vi "WVDIAL_Main2.vi"() -> ()   [LabVIEW 2012]
uses:
  WVDIAL_GlobalVariables.vi
  TypeDefinitions.llb/TypeDef_LoopStagesMain.ctl
  TypeDefinitions.llb/TypeDef_ConfigureFIleTypes.ctl
  TypeDefinitions.llb/TypeDef_MainControlSystem.ctl
  TypeDefinitions.llb/TypeDef_ChildReporting.ctl
  <vilib>/Utility/miscctls.llb/LVRectTypeDef.ctl
  <vilib>/Utility/miscctls.llb/LVPointTypeDef.ctl
panel:
  out "FileUpdateTime":dbl
  out "WritePaths":path[](array[path])
  out "FileBaseNames":string[](array[string])
  out "DataBasePath":string="C:\\Users\\h2odial\\Desktop\\WVDCode\\WVD-MCSupdate\\WVDNewArchitectureUpdate\\WVD_Architecture_Update\\DataFolder"
  out "Children Responding":T2(array[cluster])
  out "QueueElement":string
  out "LoopCounter":i32
  out "Permission Level":T3(ring)
  in  "User Comment":bool
  in  "Update Permissions":bool
  in  "Global Abort":bool
  in  "Tab Control":T4(tab)
  in  "LaserLocking":bool
  in  "MCS":bool
  in  "Weather Station":bool
  in  "Template":bool
  in  "Operations":bool
  in  "Warmup":bool
  out "error IO":errorcluster
  out "SubPanelWidth":i32
  out "SubPanelHeight":i32
  out "What to Do":string
  in  "Software Testing":bool
  out "Pages":refnum<vi>[](array[refnum])
  out "SubPanelRefs":refnum<vi>[](array[refnum])
  # "Main Programs"
  # "Testing Programs"
  # "Individual Controls"
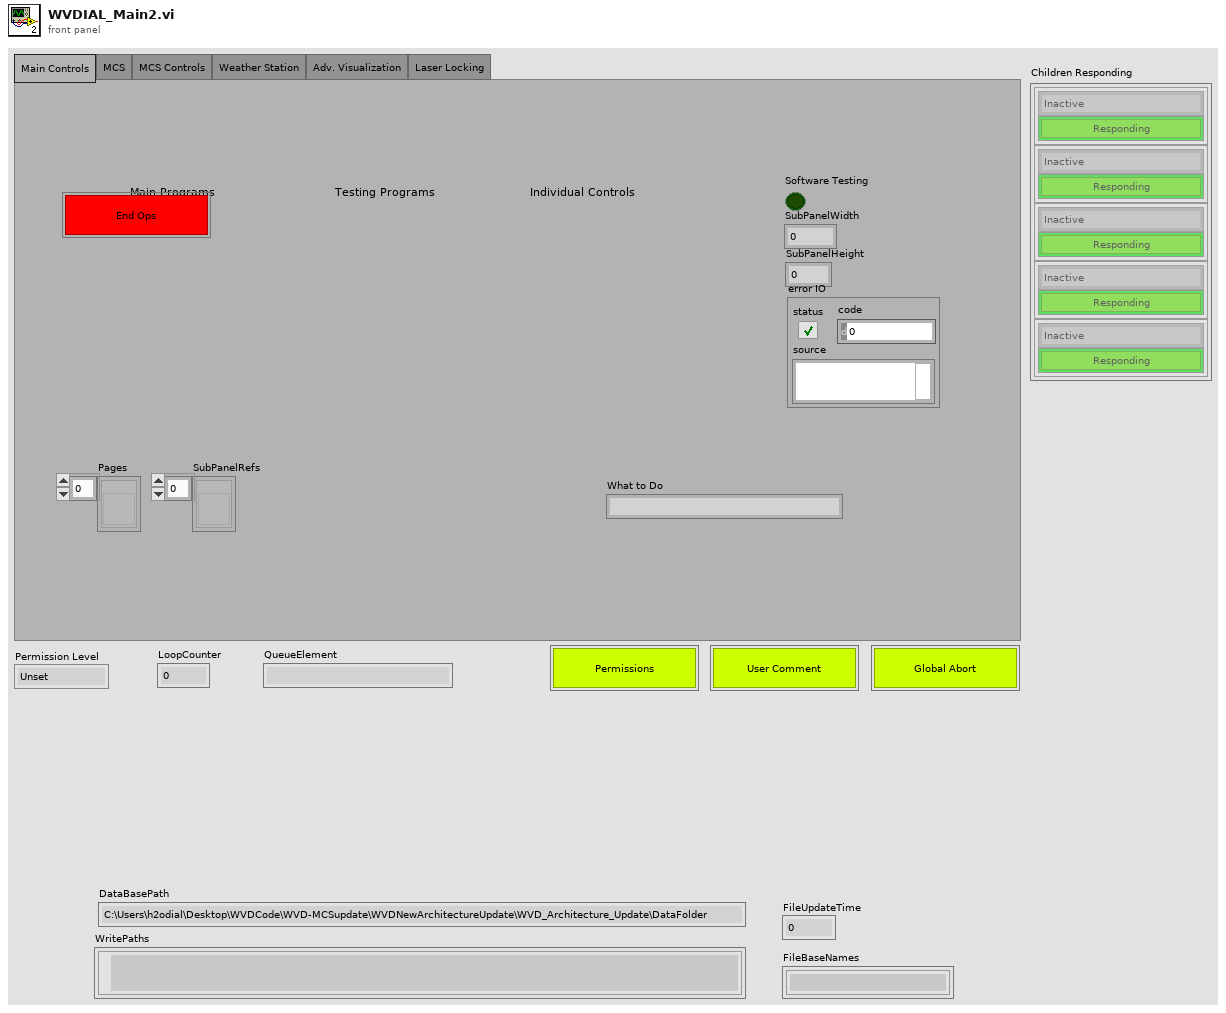
[diagram p1: front panel]
types:
  T1 = typedef "TypeDef_MainControlSystem.ctl" = enum16{"Inactive", "MCS", "MCSControls", "LaserControl", "LaserLocking", "WeatherStation", "DataDisplay", "Template", "WavelengthLocking"}
  T2 = cluster{"MainControlSystems":T1, "Responding":bool}[]
  T3 = enum16{"Unset", "Operator", "Administrator", "Full"}
  T4 = enum32{"Main Controls", "Inner Function 1", "Inner Function 2", "Inner Function 3", "Inner Function 4", "Inner Function 5", "Inner Function 6", "Inner Function 7", "Inner Function 8"}
  T5 = typedef "TypeDef_LoopStagesMain.ctl" = enum16{"Configure", "Initialize", "Idle", "ExitChildren", "Error Handler", "Exit"}
  T6 = typedef "LVPointTypeDef.ctl" = cluster{"Horizontal":i16, "Vertical":i16}
  T7 = typedef "LVRectTypeDef.ctl" = cluster{"Left":i16, "Top":i16, "Right":i16, "Bottom":i16}
  T8 = typedef "TypeDef_ConfigureFIleTypes.ctl" = enum16{"Main", "OpsMain", "OpsTemplate", "OpsWarmup", "OpsMCS", "OpsWeatherStation", "OpsWavlengthLocking", "ChildHousekeeping", "ChildLaserLocking", "ChildMCS", "ChildMCSControl", "ChildPowerSwitches", "ChildQuantumComposer", "ChildTemplate", "ChildUPS", "ChildWeatherStation", "ChildPlotting", "TestingSwitches", "TestingWavemeter"}
  T9 = typedef "TypeDef_ChildReporting.ctl" = cluster{"Child Command Stop":bool, "Child Responding":bool, "MainControlSystems":T1, "LastReportTime":dbl, "Child Exiting":bool}
  T10 = enum32{"Page Enabled", "Page Disabled", "Page Disabled & Grayed"}
  T11 = cluster{"MainControlSystems":T1, "Responding":bool}
  T12 = enum16{"Always On", "Always Off", "Off While Running"}
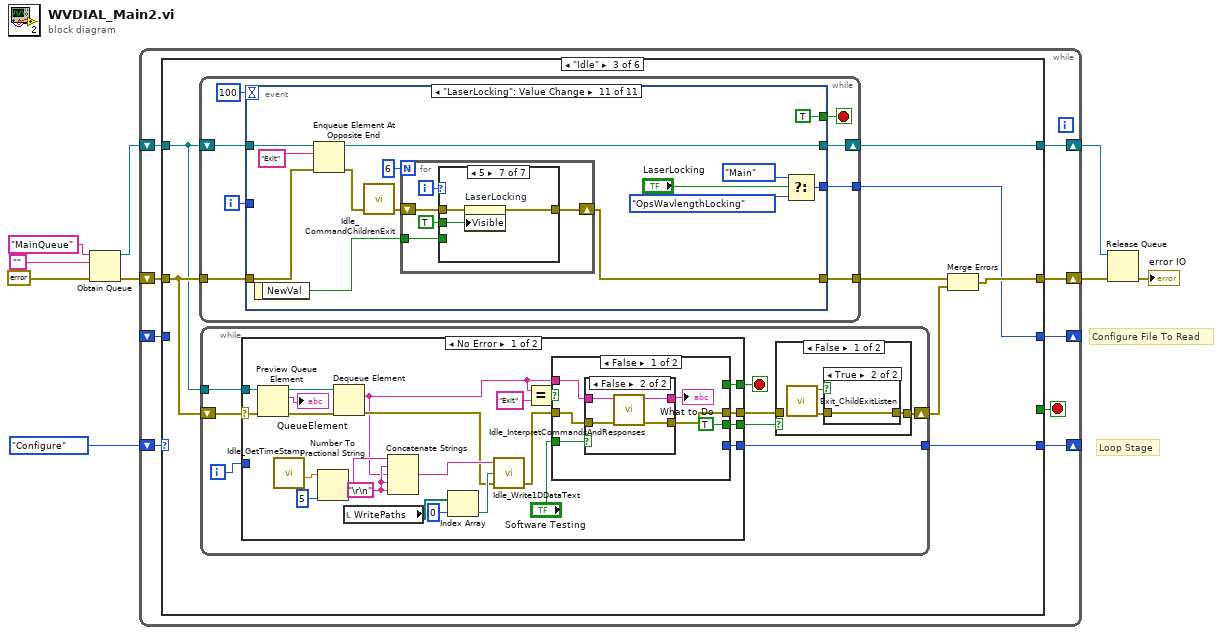
[diagram p0: block diagram]
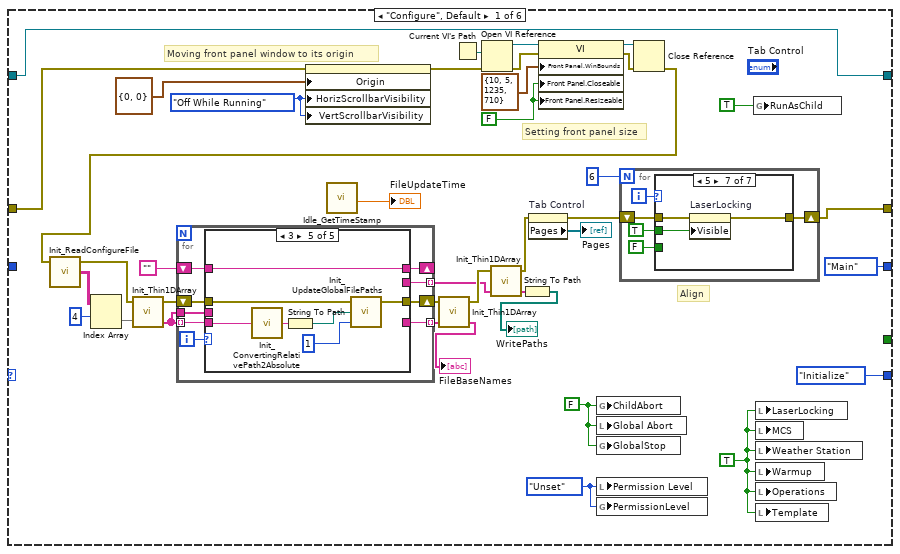
[diagram p2: hidden frame]
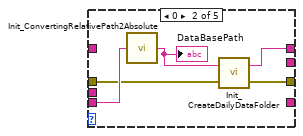
[diagram p4: hidden frame]
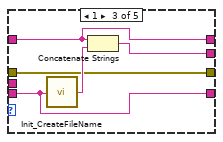
[diagram p5: hidden frame]
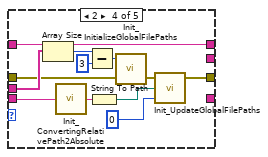
[diagram p6: hidden frame]
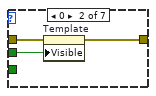
[diagram p8: hidden frame]
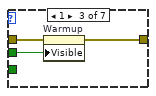
[diagram p9: hidden frame]
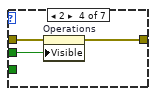
[diagram p10: hidden frame]
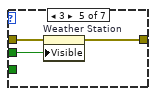
[diagram p11: hidden frame]
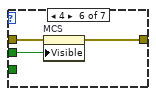
[diagram p12: hidden frame]
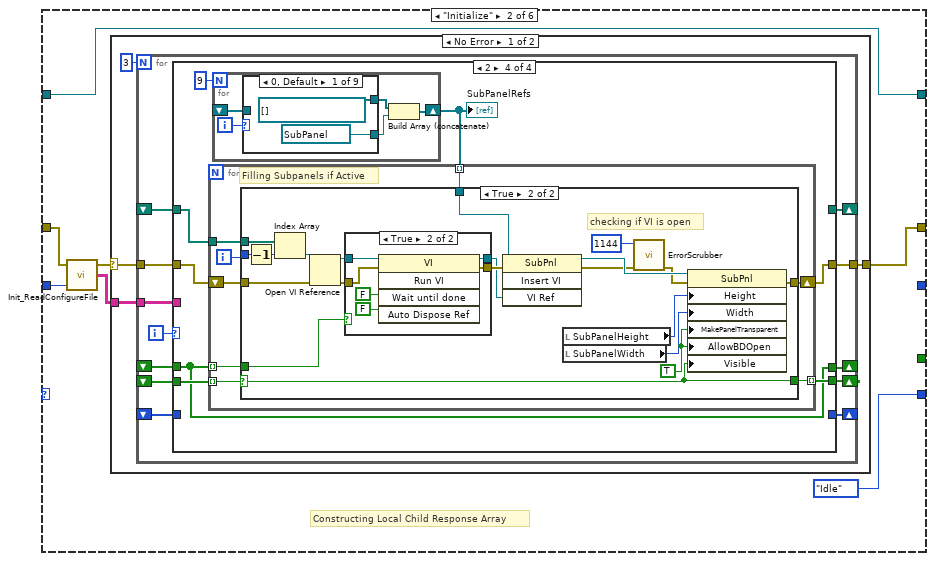
[diagram p13: hidden frame]
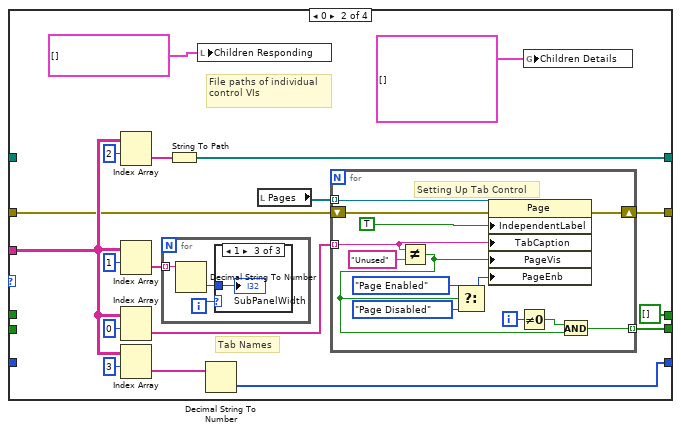
[diagram p15: hidden frame]
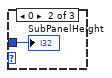
[diagram p17: hidden frame]
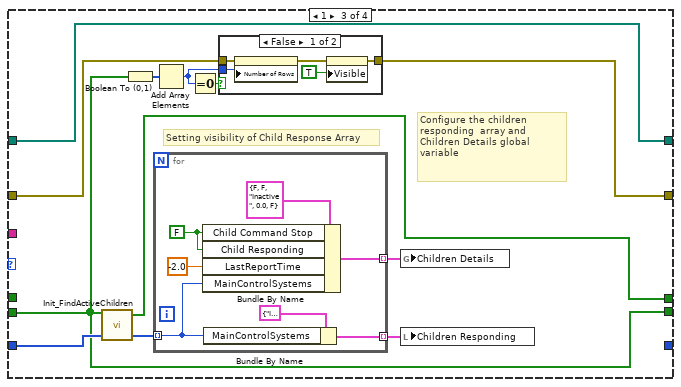
[diagram p18: hidden frame]
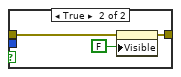
[diagram p19: hidden frame]
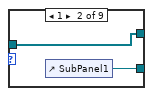
[diagram p20: hidden frame]
diagram:
  # "Configure File To Read"
  # "Loop Stage"
  n1 = Obtain Queue(name (unnamed)="MainQueue", element data type="", error in (no error)=errorcluster {"status"=FALSE, "code"=0, "source"=""}) -> (queue out=w3:refnum<queue>, error out=w4:errorcluster)  [unwired: 2 in, 1 out]
  n2 = while {
    shift-right: [w14] -> w7
    shift-left: w4 -> [w15]
    shift-right: [w13] -> w8
    shift-left: w3 -> [w12]
    shift-right: [w17] -> _
    shift-left: TypeDef_LoopStagesMain."Configure" ("Enum") -> [w18]
    shift-right: [w11] -> _
    shift-left: _ -> [w10]
    stop <- w16 stop-if-true
    n3 = case shown="\"Idle\"" w18 {
      tunnel: [TypeDef_LoopStagesMain."Initialize" ("Enum") TypeDef_LoopStagesMain."Idle" ("Enum") w288 TypeDef_LoopStagesMain."Initialize" ("Enum") TypeDef_LoopStagesMain."Idle" ("Enum") TypeDef_LoopStagesMain."Exit" ("Enum")] -> w17
      tunnel: [_ _ _ _ _ TRUE] -> w16
      tunnel: [w38 w127 w285 w646 w661 w667] -> w14
      tunnel: w15 -> [w40 w125 w289 w645 w661 w664]
      tunnel: [w41 w126 w290 w650 w659 w669] -> w13
      tunnel: w12 -> [w41 w126 w284 w650 w659 w669]
      tunnel: [TypeDef_ConfigureFIleTypes."Main" ("MainControlSystems") _ w283 w648 _ _] -> w11
      tunnel: w10 -> [_ w122 _ w648 _ _]
      frame "Configure", Default {
        w44 = T12."Off While Running" ("Vertical Scrollbar Visibility")
        w51 = FALSE
        w37 = TRUE ("Warmup")
        w52 = T3."Unset" ("Permission Level")
        w54 = FALSE ("Global Stop")
        # "Align"
        # "Setting front panel size"
        # "Moving front panel window to its origin"
        n4 = property on="Pane" class="Pane"(error in=w40, "Origin"=T6 {"Horizontal"=0, "Vertical"=0}, "HorizScrollbarVisibility"=w44, "VertScrollbarVisibility"=w44) -> (error out=w42:errorcluster)  [unwired: 1 in, 1 out]
        n5 = call "Idle_GetTimeStamp.vi"() -> ("Fractional Hours"=→"FileUpdateTime":dbl)  [unwired: 11 in]
        n6 = Current VI's Path() -> (path=w45:path)
        n7 = Open VI Reference(vi path=w45, error in (no error)=w42) -> (vi reference=w46:refnum<vi>, error out=w47:errorcluster)  [unwired: 4 in]
        n8 = property class="VI"(reference=w46, error in=w47, "Front Panel.WinBounds"=T7 {"Left"=10, "Top"=5, "Right"=1235, "Bottom"=710} ("Front Panel Window:Panel Bounds"), "Front Panel.Closeable"=w51, "Front Panel.Resizeable"=w51) -> (reference out=w48:refnum<vi>, error out=w49:errorcluster)
        n9 = global write "WVDIAL_GlobalVariables.vi" "ChildAbort"(w54) -> ()
        n10 = local write "Global Abort"(w54) -> ()
        n11 = global write "WVDIAL_GlobalVariables.vi" "GlobalStop"(w54) -> ()
        n12 = local write "Permission Level"(w52) -> ()
        n13 = global write "WVDIAL_GlobalVariables.vi" "PermissionLevel"(w52) -> ()
        n14 = Close Reference(reference=w48, error in (no error)=w49) -> (error out=w19:errorcluster)
        n15 = call "Init_ReadConfigureFile.vi"("error in"=w19) -> ("Parsed List"=w22:string[][], "error out"=w23:errorcluster)  [unwired: 2 in, 1 out]
        n16 = Index Array(array=w22, index (row)=4) -> (element=w26:string[])  [unwired: 1 in]
        n17 = call "Init_Thin1DArray.vi"("Padded Array"=w26, "ErrorIn"=w23) -> ("ThinnedArray"=w28:string[], "ErrorOut"=w27:errorcluster)  [unwired: 1 in, 1 out]
        n18 = for {
          shift-right: [w63] -> w30
          shift-left: w27 -> [w64]
          tunnel: w28 -> [w65] mode=indexing
          shift-right: [w62] -> _
          shift-left: "" -> [w61]
          tunnel: [w60] -> w31 mode=indexing
          tunnel: [w59] -> w34 mode=indexing
          tunnel: w28 -> [w58]
          i -> [w66]
          n19 = case shown="3" w66 {
            tunnel: w65 -> [_ w73 w75 w90 w97]
            tunnel: w64 -> [w67 w71 w77 w87 w95]
            tunnel: [w67 w70 w77 w86 w94] -> w63
            tunnel: [w68 w72 w76 w89 w96] -> w62
            tunnel: w61 -> [w68 _ w76 w89 w96]
            tunnel: [_ _ w75 _ _] -> w60
            tunnel: [_ _ w74 _ _] -> w59
            tunnel: w58 -> [_ _ _ w88 _]
            frame -1, Default {
            }
            frame 0 {
              n20 = call "Init_ConvertingRelativePath2Absolute.vi"("PathFromConfigureFileIn"=w73) -> ("PathOut"=w69:string)
              "DataBasePath" <- w69
              n21 = call "Init_CreateDailyDataFolder.vi"("ErrorIn"=w71, "PathIn"=w69) -> ("ErrorOut"=w70:errorcluster, "PathOut"=w72:string)
            }
            frame 1 {
              n22 = call "Init_CreateFileName.vi"("BaseFileName"=w75) -> ("FileName"=w78:string)
              n23 = Concatenate Strings(w76, w78) -> (w74:string)
            }
            frame 2 {
              n24 = Array Size(array=w88) -> (size(s)=w84:i32)
              n25 = call "Init_ConvertingRelativePath2Absolute.vi"("PathFromConfigureFileIn"=w90) -> ("PathOut"=w85:string)
              n26 = Subtract(x=w84, y=3) -> (x-y=w82:i32)
              n27 = String To Path(string=w85) -> (path=w81:path)
              n28 = call "Init_InitializeGlobalFilePaths.vi"("ErrorIn"=w87, "Entries"=w82) -> ("ErrorOut"=w80:errorcluster)  [unwired: 1 in]
              n29 = call "Init_UpdateGlobalFilePaths.vi"("PathIndex"=0, "NewPath"=w81, "ErrorIn"=w80) -> ("ErrorOut"=w86:errorcluster)  [unwired: 2 in]
            }
            frame 3 {
              n30 = call "Init_ConvertingRelativePath2Absolute.vi"("PathFromConfigureFileIn"=w97) -> ("PathOut"=w93:string)
              n31 = String To Path(string=w93) -> (path=w92:path)
              n32 = call "Init_UpdateGlobalFilePaths.vi"("PathIndex"=1, "NewPath"=w92, "ErrorIn"=w95) -> ("ErrorOut"=w94:errorcluster)  [unwired: 2 in]
            }
          }
        }
        n33 = call "Init_Thin1DArray.vi"("Padded Array"=w31, "ErrorIn"=w30) -> ("ThinnedArray"=→"FileBaseNames":string[], "ErrorOut"=w35:errorcluster)  [unwired: 1 in, 1 out]
        n34 = call "Init_Thin1DArray.vi"("Padded Array"=w34, "ErrorIn"=w35) -> ("ThinnedArray"=w32:string[], "ErrorOut"=w21:errorcluster)  [unwired: 1 in, 1 out]
        n35 = String To Path(string=w32) -> (path=→"WritePaths":path[])
        n36 = property on="Tab Control" class="TabCtl (strict)"(error in=w21) -> (error out=w39:errorcluster, "Pages"=→"Pages":refnum<vi>[])  [unwired: 1 in, 1 out]
        n37 = for {
          N: 6 -> [_]
          shift-right: [w100] -> w38
          shift-left: w39 -> [w101]
          i -> [w102]
          n38 = case shown="5" w102 {
            tunnel: w101 -> [w103 w106 w109 w112 w115 w117 w121]
            tunnel: [w103 w105 w108 w111 w114 w118 w120] -> w100
            tunnel: TRUE ("Visible") -> [_ w104 w107 w110 w113 w116 w119]
            tunnel: FALSE ("Visible") -> [_ _ _ _ _ _ _]
            frame -1, Default {
            }
            frame 0 {
              n39 = property on="Template" class="Bool (strict)"(error in=w106, "Visible"=w104) -> (error out=w105:errorcluster)  [unwired: 1 in, 1 out]
            }
            frame 1 {
              n40 = property on="Warmup" class="Bool (strict)"(error in=w109, "Visible"=w107) -> (error out=w108:errorcluster)  [unwired: 1 in, 1 out]
            }
            frame 2 {
              n41 = property on="Operations" class="Bool (strict)"(error in=w112, "Visible"=w110) -> (error out=w111:errorcluster)  [unwired: 1 in, 1 out]
            }
            frame 3 {
              n42 = property on="Weather Station" class="Bool (strict)"(error in=w115, "Visible"=w113) -> (error out=w114:errorcluster)  [unwired: 1 in, 1 out]
            }
            frame 4 {
              n43 = property on="MCS" class="Bool (strict)"(error in=w117, "Visible"=w116) -> (error out=w118:errorcluster)  [unwired: 1 in, 1 out]
            }
            frame 5 {
              n44 = property on="LaserLocking" class="Bool (strict)"(error in=w121, "Visible"=w119) -> (error out=w120:errorcluster)  [unwired: 1 in, 1 out]
            }
          }
        }
        n45 = global write "WVDIAL_GlobalVariables.vi" "RunAsChild"(TRUE ("RunAsChild")) -> ()
        n46 = local write "LaserLocking"(w37) -> ()
        n47 = local write "MCS"(w37) -> ()
        n48 = local write "Weather Station"(w37) -> ()
        n49 = local write "Warmup"(w37) -> ()
        n50 = local write "Operations"(w37) -> ()
        n51 = local write "Template"(w37) -> ()
      }
      frame "Initialize" {
        # "Constructing Local Child Response Array"
        n52 = call "Init_ReadConfigureFile.vi"("ConfigureFileType"=w122, "error in"=w125) -> ("Parsed List"=w123:string[][], "error out"=w124:errorcluster)  [unwired: 1 in, 1 out]
        n53 = case shown="No Error" w124 {
          selector: w124 -> [w131 w282]
          tunnel: [w132 w282] -> w127
          tunnel: w123 -> [w130 _]
          frame No Error {
            n54 = for {
              N: 3 -> [_]
              tunnel: [w144] -> w132
              tunnel: w131 -> [w137]
              tunnel: w130 -> [w142]
              shift-right: [w141] -> _
              shift-left: _ -> [w140]
              shift-right: [w139] -> _
              shift-left: _ -> [w138]
              shift-right: [w136] -> _
              shift-left: _ -> [w135]
              shift-right: [w134] -> _
              shift-left: _ -> [w133]
              i -> [w143]
              n55 = case shown="2" w143 {
                tunnel: [w148 w159 w194 w220] -> w144
                tunnel: w137 -> [w148 w151 w195 w217]
                tunnel: w142 -> [_ w157 _ _]
                tunnel: [w149 w163 w188 _] -> w141
                tunnel: w140 -> [w149 _ w188 w219]
                tunnel: [w147 w160 w190 w216] -> w139
                tunnel: w138 -> [w147 _ w190 w218]
                tunnel: [w146 w155 _ _] -> w136
                tunnel: w135 -> [w146 _ w191 _]
                tunnel: [w145 bool[] [] ("StartSubVI") w186 w213] -> w134
                tunnel: w133 -> [w145 _ _ w213]
                frame -1, Default {
                }
                frame 0 {
                  # "File paths of individual control VIs"
                  # "Tab Names"
                  n56 = Index Array(array=w157, index (row)=2) -> (element=w164:string[])  [unwired: 1 in]
                  n57 = Index Array(array=w157, index (row)=1) -> (element=w162:string[])  [unwired: 1 in]
                  n58 = Index Array(array=w157, index (row)=0) -> (element=w161:string[])  [unwired: 1 in]
                  n59 = Index Array(array=w157, index (row)=3) -> (element=w156:string[])  [unwired: 1 in]
                  n60 = for {
                    tunnel: w162 -> [w182] mode=indexing
                    i -> [w183]
                    n61 = Decimal String To Number(string=w182) -> (number=w181:i32)  [unwired: 2 in, 1 out]
                    n62 = case shown="1" w183 {
                      tunnel: w181 -> [_ w184 w185]
                      frame -1, Default {
                      }
                      frame 0 {
                        "SubPanelHeight" <- w184
                      }
                      frame 1 {
                        "SubPanelWidth" <- w185
                      }
                    }
                  }
                  n63 = String To Path(string=w164) -> (path=w163:path[])
                  n64 = local write "Children Responding"(T2 [] ("Children Responding")) -> ()
                  n65 = Decimal String To Number(string=w156) -> (number=w155:i32[])  [unwired: 2 in, 1 out]
                  n66 = local read "Pages"() -> (w152:refnum<vi>[])
                  n67 = for {
                    tunnel: w161 -> [w174] mode=indexing
                    tunnel: w152 -> [w177] mode=indexing
                    shift-right: [w175] -> w159
                    shift-left: w151 -> [w176]
                    tunnel: [w171] -> w160 mode=indexing
                    i -> [w172]
                    # "Setting Up Tab Control"
                    n68 = Not Equal?(x=w174, y="Unused") -> (x != y?=w169:bool)
                    n69 = Select(t=T10."Page Enabled" ("Page Enabled State"), s=w169, f=T10."Page Disabled" ("Page Enabled State")) -> (s? t:f=w168:T10)
                    n70 = property class="Page"(reference=w177, error in=w176, "IndependentLabel"=TRUE ("Independent Label"), "TabCaption"=w174, "PageVis"=w169, "PageEnb"=w168) -> (error out=w175:errorcluster)  [unwired: 1 out]
                    n71 = Not Equal To 0?(x=w172) -> (x != 0?=w173:bool)
                    n72 = And(x=w173, y=w169) -> (x .and. y?=w171:bool)
                  }
                  n73 = global write "WVDIAL_GlobalVariables.vi" "Children Details"(T9[] []) -> ()
                }
                frame 1 {
                  # "Setting visibility of Child Response Array"
                  # "Configure the children responding  array and Children Details global variable"
                  n74 = call "Init_FindActiveChildren.vi"("ChannelType"=w191, "ChannelOn"=w190) -> ("ActiveTypes"=w189:i32[], "StartSubVI"=w186:bool[])  [unwired: 1 in, 1 out]
                  n75 = Boolean To (0,1)(Boolean=w190) -> (0, 1=w197:i16[])
                  n76 = for {
                    tunnel: [w211] -> w196 mode=indexing
                    tunnel: w189 -> [w206] mode=indexing
                    tunnel: [w209] -> w187 mode=indexing
                    w208 = FALSE
                    n77 = Bundle By Name(cluster=T9 {"Child Command Stop"=FALSE, "Child Responding"=FALSE, "MainControlSystems"=enum."Inactive", "LastReportTime"=0.0, "Child Exiting"=FALSE} ("Child Details"), "Child Command Stop"=w208, "Child Responding"=w208, "LastReportTime"=-2.0, "MainControlSystems"=w206) -> (w209:T9)
                    n78 = Bundle By Name(cluster=T11 {"MainControlSystems"=enum."Inactive", "Responding"=TRUE} ("ChildResponse"), "MainControlSystems"=w206) -> (w211:T11)
                  }
                  n79 = Add Array Elements(numeric array=w197) -> (sum=w193:i16)
                  n80 = Equal To 0?(x=w193) -> (x = 0?=w192:bool)
                  n81 = case shown="False" w192 {
                    tunnel: w195 -> [w202 w205]
                    tunnel: [w199 w204] -> w194
                    tunnel: w193 -> [w201 _]
                    frame False {
                      n82 = property on="Children Responding" class="Arr (strict)"(error in=w202, "Number of Rows"=w201) -> (error out=w200:errorcluster)  [unwired: 1 in, 1 out]
                      n83 = property on="Children Responding" class="Arr (strict)"(error in=w200, "Visible"=TRUE) -> (error out=w199:errorcluster)  [unwired: 1 in, 1 out]
                    }
                    frame True {
                      n84 = property on="Children Responding" class="Arr (strict)"(error in=w205, "Visible"=FALSE) -> (error out=w204:errorcluster)  [unwired: 1 in, 1 out]
                    }
                  }
                  n85 = global write "WVDIAL_GlobalVariables.vi" "Children Details"(w187) -> ()
                  n86 = local write "Children Responding"(w196) -> ()
                }
                frame 2 {
                  n87 = for {
                    N: 9 -> [_]
                    shift-right: [w225] -> w214
                    shift-left: _ -> [w221]
                    i -> [w224]
                    n88 = case shown="0, Default" w224 {
                      tunnel: [refnum<vi> refnum ("SubPanel8") w229 w231 w233 w235 w237 w239 w241 w243] -> w223
                      tunnel: [refnum<vi>[] [] w228 w230 w232 w234 w236 w238 w240 w242] -> w222
                      tunnel: w221 -> [_ w228 w230 w232 w234 w236 w238 w240 w242]
                      frame 0, Default {
                      }
                      frame 1 {
                        n89 = control-ref of="SubPanel1"() -> (w229:refnum<vi>)
                      }
                      frame 2 {
                        n90 = control-ref of="SubPanel2"() -> (w231:refnum<vi>)
                      }
                      frame 3 {
                        n91 = control-ref of="SubPanel3"() -> (w233:refnum<vi>)
                      }
                      frame 4 {
                        n92 = control-ref of="SubPanel4"() -> (w235:refnum<vi>)
                      }
                      frame 5 {
                        n93 = control-ref of="SubPanel5"() -> (w237:refnum<vi>)
                      }
                      frame 6 {
                        n94 = control-ref of="SubPanel6"() -> (w239:refnum<vi>)
                      }
                      frame 7 {
                        n95 = control-ref of="SubPanel7"() -> (w241:refnum<vi>)
                      }
                      frame 8 {
                        n96 = control-ref of="SubPanel8"() -> (w243:refnum<vi>)
                      }
                    }
                    n97 = Build Array (concatenate)(w222, w223) -> (w225:refnum<vi>[])
                  }
                  "SubPanelRefs" <- w214
                  n98 = for {
                    shift-right: [w250] -> w220
                    shift-left: w217 -> [w251]
                    tunnel: w219 -> [w249]
                    tunnel: w218 -> [w246] mode=indexing
                    tunnel: [w248] -> w216 mode=indexing
                    tunnel: w214 -> [w245] mode=indexing
                    tunnel: w213 -> [w244] mode=indexing
                    i -> [w247]
                    # "Filling Subpanels if Active"
                    n99 = case shown="True" w246 {
                      selector: w246 -> [w252 w258]
                      tunnel: w251 -> [w253 w273]
                      tunnel: [w253 w260] -> w250
                      tunnel: w249 -> [_ w272]
                      tunnel: w247 -> [_ w264]
                      tunnel: [w252 w258] -> w248
                      tunnel: w245 -> [_ w261]
                      tunnel: w244 -> [_ w257]
                      frame False {
                      }
                      frame True {
                        w265 = TRUE ("Allow User to Open Diagram")
                        # "checking if VI is open"
                        n100 = Decrement(x=w264) -> (x-1=w263:i32)
                        n101 = Index Array(array=w272, index=w263) -> (element=w271:path)
                        n102 = Open VI Reference(vi path=w271, error in (no error)=w273) -> (vi reference=w270:refnum<vi>, error out=w269:errorcluster)  [unwired: 4 in]
                        n103 = case shown="True" w257 {
                          tunnel: w270 -> [w275 w281]
                          tunnel: w269 -> [w274 w280]
                          tunnel: [w274 w278] -> w268
                          tunnel: [w275 w276] -> w259
                          frame False {
                          }
                          frame True {
                            n104 = invoke class="VI" method="Run VI"(reference=w281, error in=w280, "Wait until done"=FALSE ("Wait Until Done"), "Auto Dispose Ref"=FALSE ("Auto Dispose Reference")) -> (reference out=w276:refnum<vi>, error out=w278:errorcluster)  [unwired: 1 in, 3 out]
                          }
                        }
                        n105 = invoke on="Invoke Node" class="SubPnl" method="Insert VI"(reference=w261, error in=w268, "VI Ref"=w259) -> (reference out=w262:refnum<vi>, error out=w255:errorcluster)  [unwired: 1 in, 2 out]
                        n106 = local read "SubPanelHeight"() -> (w267:i32)
                        n107 = local read "SubPanelWidth"() -> (w266:i32)
                        n108 = call "ErrorScrubber.vi"("error in (no error)"=w255, "y"=1144) -> ("error out"=w256:errorcluster)  [unwired: 9 in]
                        n109 = property on="Property Node" class="SubPnl"(reference=w262, error in=w256, "Height"=w267, "Width"=w266, "MakePanelTransparent"=w265, "AllowBDOpen"=w265, "Visible"=w258) -> (error out=w260:errorcluster)  [unwired: 1 out]
                      }
                    }
                  }
                }
              }
            }
          }
          frame Error {
          }
        }
      }
      frame "Idle" {
        n110 = while {
          tunnel: w289 -> [w355]
          shift-right: [w350] -> w290
          shift-left: w284 -> [w351]
          tunnel: [w349] -> w286
          tunnel: [w348] -> w283
          i -> [w352]
          stop <- w353 stop-if-true
          n111 = event shown="[10] \"LaserLocking\": Value Change" {
            selector: _ -> [_ _ _ _ _ _ _ _ _ _ _]
            dyn-events: _ -> [_ _ _ _ _ _ _ _ _ _ _]
            timeout: 100 -> [_ _ _ _ _ _ _ _ _ _ _]
            tunnel: w355 -> [w362 w364 w370 w374 w389 w427 w466 w504 w542 w580 w618]
            tunnel: [_ "Global Abort" _ _ TRUE ("Global Abort") TRUE ("Global Abort") TRUE ("Global Abort") TRUE ("Global Abort") TRUE ("Global Abort") TRUE ("Global Abort") TRUE ("Global Abort")] -> w353
            tunnel: w352 -> [w361 _ _ _ _ _ _ _ _ _ _]
            tunnel: w351 -> [w360 w367 w373 w377 w391 w429 w468 w506 w544 w582 w620]
            tunnel: [w360 w366 w372 w376 w390 w428 w467 w505 w543 w581 w619] -> w350
            tunnel: [w362 w363 w369 w375 w380 w419 w460 w498 w536 w574 w612] -> w349
            tunnel: [_ _ _ _ w392 w430 w458 w496 w534 w572 w610] -> w348
            event Timeout {
              n112 = event-data() -> ()  [unwired: 1 in, 1 out]
              n113 = global read "WVDIAL_GlobalVariables.vi" "PermissionLevel"() -> (→"Permission Level":i32)
              n114 = local read "Children Responding"() -> (w357:T2)
              n115 = call "Idle_MainIdleProcess.vi"("ChildrenResponding"=w357) -> ("ChildrenDetailsUpdated"=w359:T9[], "ChildrenResponding"=→"Children Responding":T2)  [unwired: 1 in]
              n116 = global write "WVDIAL_GlobalVariables.vi" "Children Details"(w359) -> ()
              "LoopCounter" <- w361
            }
            event "Global Abort": Value Change {
              n117 = event-data() -> ()  [unwired: 1 in, 1 out]
              n118 = Enqueue Element At Opposite End(queue=w367, element="Exit", error in (no error)=w364) -> (queue out=w366:refnum<queue>, error out=w363:errorcluster)  [unwired: 1 in, 1 out]
              n119 = global write "WVDIAL_GlobalVariables.vi" "GlobalStop"("Global Abort") -> ()
            }
            event "Update Permissions": Value Change {
              n120 = event-data() -> ()  [unwired: 1 in, 1 out]
              n121 = Enqueue Element(queue=w373, element="System_OpenPermissionsVI", error in (no error)=w370) -> (queue out=w372:refnum<queue>, error out=w369:errorcluster)  [unwired: 1 in, 1 out]
            }
            event "User Comment": Value Change {
              n122 = event-data() -> ()  [unwired: 1 in, 1 out]
              n123 = Enqueue Element(queue=w377, element="System_OpenUserCommentVI", error in (no error)=w374) -> (queue out=w376:refnum<queue>, error out=w375:errorcluster)  [unwired: 1 in, 1 out]
            }
            event "Template": Value Change {
              n124 = event-data() -> ("NewVal"=w379:bool)  [unwired: 1 in]
              n125 = Enqueue Element At Opposite End(queue=w391, element="Exit", error in (no error)=w389) -> (queue out=w390:refnum<queue>, error out=w384:errorcluster)  [unwired: 1 in, 1 out]
              n126 = call "Idle_CommandChildrenExit.vi"("ErrorIn"=w384) -> ("ErrorOut"=w381:errorcluster)  [unwired: 4 in]
              n127 = for {
                N: 6 -> [_]
                shift-right: [w395] -> w380
                shift-left: w381 -> [w396]
                tunnel: w379 -> [w393]
                i -> [w397]
                n128 = case shown="0" w397 {
                  tunnel: w396 -> [w398 w401 w404 w407 w410 w412 w416]
                  tunnel: [w398 w400 w403 w406 w409 w413 w415] -> w395
                  tunnel: TRUE ("Visible") -> [_ w399 _ _ _ _ _]
                  tunnel: w393 -> [_ _ w402 w405 w408 w411 w414]
                  frame -1, Default {
                  }
                  frame 0 {
                    n129 = property on="Template" class="Bool (strict)"(error in=w401, "Visible"=w399) -> (error out=w400:errorcluster)  [unwired: 1 in, 1 out]
                  }
                  frame 1 {
                    n130 = property on="Warmup" class="Bool (strict)"(error in=w404, "Visible"=w402) -> (error out=w403:errorcluster)  [unwired: 1 in, 1 out]
                  }
                  frame 2 {
                    n131 = property on="Operations" class="Bool (strict)"(error in=w407, "Visible"=w405) -> (error out=w406:errorcluster)  [unwired: 1 in, 1 out]
                  }
                  frame 3 {
                    n132 = property on="Weather Station" class="Bool (strict)"(error in=w410, "Visible"=w408) -> (error out=w409:errorcluster)  [unwired: 1 in, 1 out]
                  }
                  frame 4 {
                    n133 = property on="MCS" class="Bool (strict)"(error in=w412, "Visible"=w411) -> (error out=w413:errorcluster)  [unwired: 1 in, 1 out]
                  }
                  frame 5 {
                    n134 = property on="LaserLocking" class="Bool (strict)"(error in=w416, "Visible"=w414) -> (error out=w415:errorcluster)  [unwired: 1 in, 1 out]
                  }
                }
              }
              n135 = Select(t=TypeDef_ConfigureFIleTypes."Main" ("MainControlSystems"), s="Template", f=TypeDef_ConfigureFIleTypes."OpsTemplate" ("MainControlSystems")) -> (s? t:f=w392:T8)
            }
            event "Warmup": Value Change {
              n136 = event-data() -> ("NewVal"=w418:bool)  [unwired: 1 in]
              n137 = Enqueue Element At Opposite End(queue=w429, element="Exit", error in (no error)=w427) -> (queue out=w428:refnum<queue>, error out=w423:errorcluster)  [unwired: 1 in, 1 out]
              n138 = call "Idle_CommandChildrenExit.vi"("ErrorIn"=w423) -> ("ErrorOut"=w420:errorcluster)  [unwired: 4 in]
              n139 = for {
                N: 6 -> [_]
                shift-right: [w433] -> w419
                shift-left: w420 -> [w434]
                tunnel: w418 -> [w431]
                i -> [w435]
                n140 = case shown="5" w435 {
                  tunnel: w434 -> [w436 w439 w442 w445 w448 w450 w454]
                  tunnel: [w436 w438 w441 w444 w447 w451 w453] -> w433
                  tunnel: TRUE ("Visible") -> [_ _ w440 _ _ _ _]
                  tunnel: w431 -> [_ w437 _ w443 w446 w449 w452]
                  frame -1, Default {
                  }
                  frame 0 {
                    n141 = property on="Template" class="Bool (strict)"(error in=w439, "Visible"=w437) -> (error out=w438:errorcluster)  [unwired: 1 in, 1 out]
                  }
                  frame 1 {
                    n142 = property on="Warmup" class="Bool (strict)"(error in=w442, "Visible"=w440) -> (error out=w441:errorcluster)  [unwired: 1 in, 1 out]
                  }
                  frame 2 {
                    n143 = property on="Operations" class="Bool (strict)"(error in=w445, "Visible"=w443) -> (error out=w444:errorcluster)  [unwired: 1 in, 1 out]
                  }
                  frame 3 {
                    n144 = property on="Weather Station" class="Bool (strict)"(error in=w448, "Visible"=w446) -> (error out=w447:errorcluster)  [unwired: 1 in, 1 out]
                  }
                  frame 4 {
                    n145 = property on="MCS" class="Bool (strict)"(error in=w450, "Visible"=w449) -> (error out=w451:errorcluster)  [unwired: 1 in, 1 out]
                  }
                  frame 5 {
                    n146 = property on="LaserLocking" class="Bool (strict)"(error in=w454, "Visible"=w452) -> (error out=w453:errorcluster)  [unwired: 1 in, 1 out]
                  }
                }
              }
              n147 = Select(t=TypeDef_ConfigureFIleTypes."Main" ("MainControlSystems"), s="Warmup", f=TypeDef_ConfigureFIleTypes."OpsWarmup" ("MainControlSystems")) -> (s? t:f=w430:T8)
            }
            event "Operations": Value Change {
              n148 = event-data() -> ("NewVal"=w459:bool)  [unwired: 1 in]
              n149 = Enqueue Element At Opposite End(queue=w468, element="Exit", error in (no error)=w466) -> (queue out=w467:refnum<queue>, error out=w464:errorcluster)  [unwired: 1 in, 1 out]
              n150 = call "Idle_CommandChildrenExit.vi"("ErrorIn"=w464) -> ("ErrorOut"=w461:errorcluster)  [unwired: 4 in]
              n151 = for {
                N: 6 -> [_]
                shift-right: [w471] -> w460
                shift-left: w461 -> [w472]
                tunnel: w459 -> [w469]
                i -> [w473]
                n152 = case shown="5" w473 {
                  tunnel: w472 -> [w474 w477 w480 w483 w486 w488 w492]
                  tunnel: [w474 w476 w479 w482 w485 w489 w491] -> w471
                  tunnel: TRUE ("Visible") -> [_ _ _ w481 _ _ _]
                  tunnel: w469 -> [_ w475 w478 _ w484 w487 w490]
                  frame -1, Default {
                  }
                  frame 0 {
                    n153 = property on="Template" class="Bool (strict)"(error in=w477, "Visible"=w475) -> (error out=w476:errorcluster)  [unwired: 1 in, 1 out]
                  }
                  frame 1 {
                    n154 = property on="Warmup" class="Bool (strict)"(error in=w480, "Visible"=w478) -> (error out=w479:errorcluster)  [unwired: 1 in, 1 out]
                  }
                  frame 2 {
                    n155 = property on="Operations" class="Bool (strict)"(error in=w483, "Visible"=w481) -> (error out=w482:errorcluster)  [unwired: 1 in, 1 out]
                  }
                  frame 3 {
                    n156 = property on="Weather Station" class="Bool (strict)"(error in=w486, "Visible"=w484) -> (error out=w485:errorcluster)  [unwired: 1 in, 1 out]
                  }
                  frame 4 {
                    n157 = property on="MCS" class="Bool (strict)"(error in=w488, "Visible"=w487) -> (error out=w489:errorcluster)  [unwired: 1 in, 1 out]
                  }
                  frame 5 {
                    n158 = property on="LaserLocking" class="Bool (strict)"(error in=w492, "Visible"=w490) -> (error out=w491:errorcluster)  [unwired: 1 in, 1 out]
                  }
                }
              }
              n159 = Select(t=TypeDef_ConfigureFIleTypes."Main" ("MainControlSystems"), s="Operations", f=TypeDef_ConfigureFIleTypes."OpsMain" ("MainControlSystems")) -> (s? t:f=w458:T8)
            }
            event "Weather Station": Value Change {
              n160 = event-data() -> ("NewVal"=w497:bool)  [unwired: 1 in]
              n161 = Enqueue Element At Opposite End(queue=w506, element="Exit", error in (no error)=w504) -> (queue out=w505:refnum<queue>, error out=w502:errorcluster)  [unwired: 1 in, 1 out]
              n162 = call "Idle_CommandChildrenExit.vi"("ErrorIn"=w502) -> ("ErrorOut"=w499:errorcluster)  [unwired: 4 in]
              n163 = for {
                N: 6 -> [_]
                shift-right: [w509] -> w498
                shift-left: w499 -> [w510]
                tunnel: w497 -> [w507]
                i -> [w511]
                n164 = case shown="5" w511 {
                  tunnel: w510 -> [w512 w515 w518 w521 w524 w526 w530]
                  tunnel: [w512 w514 w517 w520 w523 w527 w529] -> w509
                  tunnel: TRUE ("Visible") -> [_ _ _ _ w522 _ _]
                  tunnel: w507 -> [_ w513 w516 w519 _ w525 w528]
                  frame -1, Default {
                  }
                  frame 0 {
                    n165 = property on="Template" class="Bool (strict)"(error in=w515, "Visible"=w513) -> (error out=w514:errorcluster)  [unwired: 1 in, 1 out]
                  }
                  frame 1 {
                    n166 = property on="Warmup" class="Bool (strict)"(error in=w518, "Visible"=w516) -> (error out=w517:errorcluster)  [unwired: 1 in, 1 out]
                  }
                  frame 2 {
                    n167 = property on="Operations" class="Bool (strict)"(error in=w521, "Visible"=w519) -> (error out=w520:errorcluster)  [unwired: 1 in, 1 out]
                  }
                  frame 3 {
                    n168 = property on="Weather Station" class="Bool (strict)"(error in=w524, "Visible"=w522) -> (error out=w523:errorcluster)  [unwired: 1 in, 1 out]
                  }
                  frame 4 {
                    n169 = property on="MCS" class="Bool (strict)"(error in=w526, "Visible"=w525) -> (error out=w527:errorcluster)  [unwired: 1 in, 1 out]
                  }
                  frame 5 {
                    n170 = property on="LaserLocking" class="Bool (strict)"(error in=w530, "Visible"=w528) -> (error out=w529:errorcluster)  [unwired: 1 in, 1 out]
                  }
                }
              }
              n171 = Select(t=TypeDef_ConfigureFIleTypes."Main" ("MainControlSystems"), s="Weather Station", f=TypeDef_ConfigureFIleTypes."OpsWeatherStation" ("MainControlSystems")) -> (s? t:f=w496:T8)
            }
            event "MCS": Value Change {
              # "Align"
              n172 = event-data() -> ("NewVal"=w535:bool)  [unwired: 1 in]
              n173 = Enqueue Element At Opposite End(queue=w544, element="Exit", error in (no error)=w542) -> (queue out=w543:refnum<queue>, error out=w540:errorcluster)  [unwired: 1 in, 1 out]
              n174 = call "Idle_CommandChildrenExit.vi"("ErrorIn"=w540) -> ("ErrorOut"=w537:errorcluster)  [unwired: 4 in]
              n175 = for {
                N: 6 -> [_]
                shift-right: [w547] -> w536
                shift-left: w537 -> [w548]
                tunnel: w535 -> [w545]
                i -> [w549]
                n176 = case shown="4" w549 {
                  tunnel: w548 -> [w550 w553 w556 w559 w562 w564 w568]
                  tunnel: [w550 w552 w555 w558 w561 w565 w567] -> w547
                  tunnel: TRUE ("Visible") -> [_ _ _ _ _ w563 _]
                  tunnel: w545 -> [_ w551 w554 w557 w560 _ w566]
                  frame -1, Default {
                  }
                  frame 0 {
                    n177 = property on="Template" class="Bool (strict)"(error in=w553, "Visible"=w551) -> (error out=w552:errorcluster)  [unwired: 1 in, 1 out]
                  }
                  frame 1 {
                    n178 = property on="Warmup" class="Bool (strict)"(error in=w556, "Visible"=w554) -> (error out=w555:errorcluster)  [unwired: 1 in, 1 out]
                  }
                  frame 2 {
                    n179 = property on="Operations" class="Bool (strict)"(error in=w559, "Visible"=w557) -> (error out=w558:errorcluster)  [unwired: 1 in, 1 out]
                  }
                  frame 3 {
                    n180 = property on="Weather Station" class="Bool (strict)"(error in=w562, "Visible"=w560) -> (error out=w561:errorcluster)  [unwired: 1 in, 1 out]
                  }
                  frame 4 {
                    n181 = property on="MCS" class="Bool (strict)"(error in=w564, "Visible"=w563) -> (error out=w565:errorcluster)  [unwired: 1 in, 1 out]
                  }
                  frame 5 {
                    n182 = property on="LaserLocking" class="Bool (strict)"(error in=w568, "Visible"=w566) -> (error out=w567:errorcluster)  [unwired: 1 in, 1 out]
                  }
                }
              }
              n183 = Select(t=TypeDef_ConfigureFIleTypes."Main" ("MainControlSystems"), s="MCS", f=TypeDef_ConfigureFIleTypes."OpsMCS" ("MainControlSystems")) -> (s? t:f=w534:T8)
            }
            event "Software Testing": Value Change {
              # "Used for aligning other cases and replicating them easily"
              # "Align"
              # "Align"
              n184 = event-data() -> ("NewVal"=w573:bool)  [unwired: 1 in]
              n185 = Enqueue Element At Opposite End(queue=w582, element="Exit", error in (no error)=w580) -> (queue out=w581:refnum<queue>, error out=w578:errorcluster)  [unwired: 1 in, 1 out]
              n186 = call "Idle_CommandChildrenExit.vi"("ErrorIn"=w578) -> ("ErrorOut"=w575:errorcluster)  [unwired: 4 in]
              n187 = for {
                N: 6 -> [_]
                shift-right: [w585] -> w574
                shift-left: w575 -> [w586]
                tunnel: w573 -> [w583]
                i -> [w587]
                n188 = case shown="0" w587 {
                  tunnel: w586 -> [w588 w591 w594 w597 w600 w602 w606]
                  tunnel: [w588 w590 w593 w596 w599 w603 w605] -> w585
                  tunnel: TRUE ("Visible") -> [_ _ _ _ _ _ _]
                  tunnel: w583 -> [_ w589 w592 w595 w598 w601 w604]
                  frame -1, Default {
                  }
                  frame 0 {
                    n189 = property on="Template" class="Bool (strict)"(error in=w591, "Visible"=w589) -> (error out=w590:errorcluster)  [unwired: 1 in, 1 out]
                  }
                  frame 1 {
                    n190 = property on="Warmup" class="Bool (strict)"(error in=w594, "Visible"=w592) -> (error out=w593:errorcluster)  [unwired: 1 in, 1 out]
                  }
                  frame 2 {
                    n191 = property on="Operations" class="Bool (strict)"(error in=w597, "Visible"=w595) -> (error out=w596:errorcluster)  [unwired: 1 in, 1 out]
                  }
                  frame 3 {
                    n192 = property on="Weather Station" class="Bool (strict)"(error in=w600, "Visible"=w598) -> (error out=w599:errorcluster)  [unwired: 1 in, 1 out]
                  }
                  frame 4 {
                    n193 = property on="MCS" class="Bool (strict)"(error in=w602, "Visible"=w601) -> (error out=w603:errorcluster)  [unwired: 1 in, 1 out]
                  }
                  frame 5 {
                    n194 = property on="LaserLocking" class="Bool (strict)"(error in=w606, "Visible"=w604) -> (error out=w605:errorcluster)  [unwired: 1 in, 1 out]
                  }
                }
              }
              n195 = Select(t=TypeDef_ConfigureFIleTypes."Main" ("MainControlSystems"), s=TRUE, f=TypeDef_ConfigureFIleTypes."OpsWarmup" ("MainControlSystems")) -> (s? t:f=w572:T8)
            }
            event "LaserLocking": Value Change {
              n196 = event-data() -> ("NewVal"=w611:bool)  [unwired: 1 in]
              n197 = Enqueue Element At Opposite End(queue=w620, element="Exit", error in (no error)=w618) -> (queue out=w619:refnum<queue>, error out=w616:errorcluster)  [unwired: 1 in, 1 out]
              n198 = call "Idle_CommandChildrenExit.vi"("ErrorIn"=w616) -> ("ErrorOut"=w613:errorcluster)  [unwired: 4 in]
              n199 = for {
                N: 6 -> [_]
                shift-right: [w623] -> w612
                shift-left: w613 -> [w624]
                tunnel: w611 -> [w621]
                i -> [w625]
                n200 = case shown="5" w625 {
                  tunnel: w624 -> [w626 w629 w632 w635 w638 w640 w644]
                  tunnel: [w626 w628 w631 w634 w637 w641 w643] -> w623
                  tunnel: TRUE ("Visible") -> [_ _ _ _ _ _ w642]
                  tunnel: w621 -> [_ w627 w630 w633 w636 w639 _]
                  frame -1, Default {
                  }
                  frame 0 {
                    n201 = property on="Template" class="Bool (strict)"(error in=w629, "Visible"=w627) -> (error out=w628:errorcluster)  [unwired: 1 in, 1 out]
                  }
                  frame 1 {
                    n202 = property on="Warmup" class="Bool (strict)"(error in=w632, "Visible"=w630) -> (error out=w631:errorcluster)  [unwired: 1 in, 1 out]
                  }
                  frame 2 {
                    n203 = property on="Operations" class="Bool (strict)"(error in=w635, "Visible"=w633) -> (error out=w634:errorcluster)  [unwired: 1 in, 1 out]
                  }
                  frame 3 {
                    n204 = property on="Weather Station" class="Bool (strict)"(error in=w638, "Visible"=w636) -> (error out=w637:errorcluster)  [unwired: 1 in, 1 out]
                  }
                  frame 4 {
                    n205 = property on="MCS" class="Bool (strict)"(error in=w640, "Visible"=w639) -> (error out=w641:errorcluster)  [unwired: 1 in, 1 out]
                  }
                  frame 5 {
                    n206 = property on="LaserLocking" class="Bool (strict)"(error in=w644, "Visible"=w642) -> (error out=w643:errorcluster)  [unwired: 1 in, 1 out]
                  }
                }
              }
              n207 = Select(t=TypeDef_ConfigureFIleTypes."Main" ("MainControlSystems"), s="LaserLocking", f=TypeDef_ConfigureFIleTypes."OpsWavlengthLocking" ("MainControlSystems")) -> (s? t:f=w610:T8)
            }
          }
        }
        n208 = while {
          tunnel: w284 -> [w297]
          tunnel: [w296] -> w288
          shift-right: [w293] -> w287
          shift-left: w289 -> [w298]
          i -> [w295]
          stop <- w294 stop-if-true
          n209 = case shown="No Error" w298 {
            selector: w298 -> [w325 w347]
            tunnel: w297 -> [w324 _]
            tunnel: [w320 _] -> w294
            tunnel: [w319 _] -> w296
            tunnel: [w318 w347] -> w292
            tunnel: w295 -> [_ _]
            tunnel: [w316 TRUE ("GlobalStop")] -> w291
            frame No Error {
              w312 = "\r\n"
              n210 = Preview Queue Element(queue=w324, error in (no error)=w325) -> (queue out=w327:refnum<queue>, element=→"QueueElement":string, error out=w326:errorcluster)  [unwired: 1 in, 1 out]
              n211 = call "Idle_GetTimeStamp.vi"() -> ("Fractional Hours"=w314:dbl)  [unwired: 11 in]
              n212 = Number To Fractional String(number=w314, precision (6)=i16 5 ("width (-)")) -> (F-format string=w313:string)  [unwired: 2 in]
              n213 = Dequeue Element(queue=w327, error in (no error)=w326) -> (element=w306:string, error out=w307:errorcluster)  [unwired: 1 in, 2 out]
              n214 = local read "WritePaths"() -> (w311:path[])
              n215 = Concatenate Strings(w313, w312, w306, w312, w312) -> (w309:string)
              n216 = Index Array(array=w311, index=0) -> (element=w308:path)
              n217 = call "Idle_Write1DDataText.vi"("ErrorIn"=w307, "Write FilePath"=w308, "Data2Write"=w309) -> ("ErrorOut"=w305:errorcluster)  [unwired: 2 in]
              n218 = Equal?(x=w306, y="Exit") -> (x = y?=w321:bool)
              n219 = case shown="False" w321 {
                tunnel: w305 -> [w333 w341]
                tunnel: w306 -> [w330 _]
                tunnel: [_ TRUE] -> w320
                tunnel: [_ w342] -> w319
                tunnel: [w332 w341] -> w318
                tunnel: "Software Testing" -> [w329 _]
                tunnel: [TRUE ("GlobalStop") w340] -> w316
                frame False {
                  n220 = case shown="False" w329 {
                    tunnel: w333 -> [w335 w339]
                    tunnel: [w335 w338] -> w332
                    tunnel: w330 -> [_ w337]
                    tunnel: ["" w336] -> w331
                    frame True {
                    }
                    frame False {
                      n221 = call "Idle_InterpretCommandsAndResponses.vi"("error in"=w339, "Input Command"=w337) -> ("error out"=w338:errorcluster, "What to Do"=w336:string)  [unwired: 6 in, 2 out]
                    }
                  }
                  "What to Do" <- w331
                }
                frame True {
                  n222 = global read "WVDIAL_GlobalVariables.vi" "GlobalStop"() -> (w340:bool)
                  n223 = Select(t=TypeDef_LoopStagesMain."Exit" ("Enum"), s=w340, f=TypeDef_LoopStagesMain."ExitChildren" ("Enum")) -> (s? t:f=w342:T5)
                }
              }
            }
            frame Error {
            }
          }
          n224 = case shown="False" w291 {
            tunnel: w292 -> [_ w304]
            tunnel: [w301 w304] -> w293
            frame False {
              n225 = call "Exit_ChildExitListen.vi"() -> ("ErrorOut"=w300:errorcluster, "TimedOut"=w299:bool)  [unwired: 10 in]
              n226 = case shown="True" w299 {
                tunnel: w300 -> [w302 w303]
                tunnel: [w302 w303] -> w301
                frame False {
                }
                frame True {
                }
              }
            }
            frame True {
            }
          }
        }
        n227 = Merge Errors(w286, w287) -> (w285:errorcluster)
      }
      frame "ExitChildren" {
        n228 = local read "SubPanelRefs"() -> (w647:refnum<vi>[])
        n229 = for {
          tunnel: w647 -> [w651] mode=indexing
          shift-right: [w654] -> w646
          shift-left: w645 -> [w653]
          # "Removing subVIs\nfrom subPanels"
          n230 = Not A Number/Path/Refnum?(number/path/refnum=w651) -> (NaN/Path/Refnum?=w652:bool)
          n231 = case shown="False" w652 {
            tunnel: w651 -> [w657 _]
            tunnel: [w656 w658] -> w654
            tunnel: w653 -> [w655 w658]
            frame False {
              n232 = invoke class="SubPnl" method="Remove VI"(reference=w657, error in=w655) -> (error out=w656:errorcluster)  [unwired: 1 in, 2 out]
            }
            frame True {
            }
          }
        }
      }
      frame "Error Handler" {
      }
      frame "Exit" {
        w663 = T3."Unset" ("Permission Level")
        w662 = FALSE ("RunAsChild")
        n233 = global write "WVDIAL_GlobalVariables.vi" "RunAsChild"(w662) -> ()
        n234 = global write "WVDIAL_GlobalVariables.vi" "ChildAbort"(w662) -> ()
        n235 = local write "Permission Level"(w663) -> ()
        n236 = global write "WVDIAL_GlobalVariables.vi" "PermissionLevel"(w663) -> ()
        n237 = local read "Pages"() -> (w665:refnum<vi>[])
        n238 = for {
          shift-right: [w673] -> w668
          shift-left: w664 -> [w677]
          tunnel: w665 -> [w676] mode=indexing
          n239 = property class="Page"(reference=w676, error in=w677, "PageVis"=TRUE ("Page Visible")) -> (reference out=w672:refnum<vi>, error out=w674:errorcluster)
          n240 = Close Reference(reference=w672, error in (no error)=w674) -> (error out=w673:errorcluster)
        }
        n241 = property on="Children Responding" class="Arr (strict)"(error in=w668, "Visible"=TRUE) -> (error out=w667:errorcluster)  [unwired: 1 in, 1 out]
      }
    }
  }
  n242 = Release Queue(queue=w8, error in (no error)=w7) -> (error out=→"error IO":errorcluster)  [unwired: 1 in, 2 out]
